vi "Scale Cell Voltage.vi"(11 "Numeric in":u8) -> (3 "Numeric out":dbl)   [LabVIEW 2014]
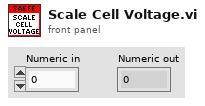
[diagram p1: front panel]
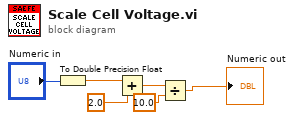
[diagram p0: block diagram]
diagram:
  n1 = To Double Precision Float(number="Numeric in") -> (double precision float=w1:dbl)
  n2 = Add(x=w1, y=2.0) -> (x+y=w4:dbl)
  n3 = Divide(x=w4, y=10.0) -> (x/y=→"Numeric out":dbl)
